vi "LSX Wait For Axis Stop.vi"(7 "pbATimeout":i32, 8 "error in (no error)":errorcluster, 9 "lATimeoutValue":i32, 10 "lAFlags":i32, 11 "lLSID":i32) -> (0 "error out":errorcluster, 3 "function return":i32, 5 "pbATimeout out":i32)   [LabVIEW 2016, in "Tango_DLL.lvlib"]
doc: "TANGOAPI int TANGOCALL LSX_WaitForAxisStop (int lLSID, int lAFlags, int lATimeoutValue, BOOL *pbATimeout);"
uses:
  Tango_DLL.lvlib
  2017/Microscope Control/Device Library/Stages/Marzhauser/SCAN IM 120 x 80/Tango DLL VIs/Tango_DLL.dll
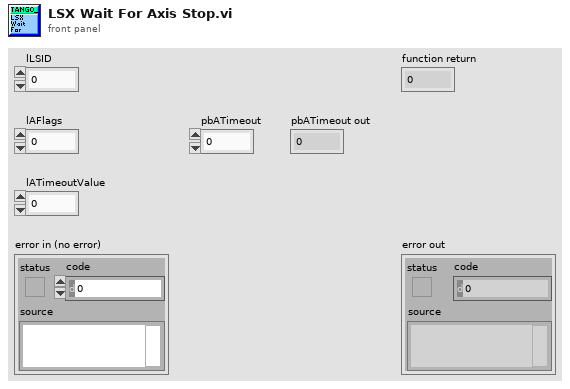
[diagram p1: front panel]
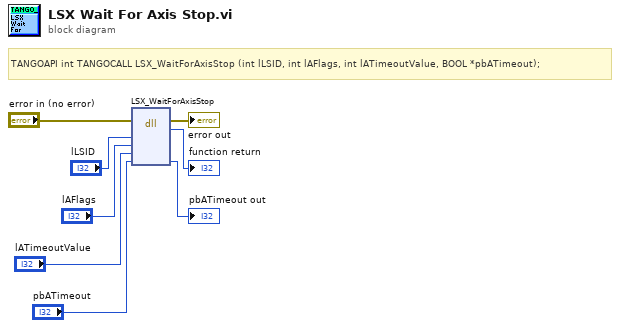
[diagram p0: block diagram]
diagram:
  # "TANGOAPI int TANGOCALL LSX_WaitForAxisStop (int lLSID, int lAFlags, int lATimeoutValue, BOOL *pbATimeout);"
  n1 = dll-call lib="C:/Users/4PiSMS/Documents/Microscope Control/2017/Microscope Control/Device Library/Stages/Marzhauser/SCAN IM 120 x 80/Tango DLL VIs/Tango_DLL.*" fn="LSX_WaitForAxisStop"(error in="error in (no error)", "lLSID"="lLSID", "lAFlags"="lAFlags", "lATimeoutValue"="lATimeoutValue", "pbATimeout"="pbATimeout") -> (error out=→"error out":errorcluster, →"function return":i32, "pbATimeout"=→"pbATimeout out":i32)  [unwired: 5 in, 1 out]
